vi "unphuck.vi"() -> ()   [LabVIEW 2009]
uses:
  <instrlib>/niScope/Controls/niScope vertical coupling.ctl
  Pulse Acquisition Method.ctl
  Pulse Queues.ctl
  <vilib>/Utility/file.llb/Write To Spreadsheet File (DBL).vi
  <instrlib>/niScope/Controls/niScope trigger slope.ctl
  <instrlib>/niScope/Controls/niScope trigger source.ctl
  <instrlib>/niScope/Configure/Trigger/niScope Configure Trigger Edge.vi
  <instrlib>/niScope/Acquire/Fetch/niScope Multi Fetch WDT.vi
panel:
  out "Number of Aquisitions":i32
  in  "Memory Repetition Period":dbl[unit]=0.025
  in  "Memory Acquisition Trigger Delay":dbl[unit] format="%.2f"
  out "Display Plot":bool
  in  "Get Reference Pulse":bool
  in  "Record Pulses":bool
  in  "Vertical range (0 to 10V)":dbl[unit]=0.01 caption="Vertical Range (V)" format="%.2f"
  in  "Desired Sample Rate":dbl[unit]=100000000.0 caption="Min. Sample Rate" step=1.0 format="%.2p"
  in  "Vertical coupling":T1 caption="Vertical Coupling" items=["AC", "DC", "Ground"]
  in  "Acquisition Time per Pulse":dbl[unit]=9.999999999999999e-06 format="%#.2g"
  out "Fetches Remaining":i32 caption="Number of Runs"
  out "Actual Sample Rate":dbl[unit]
  out "Number of Samples per Pulse":i32
  out "Acquisition Sequence":dbl[](graph)
  out "Total Acquired Time":dbl[unit]
  out "Total Number of Datapoints":i64=1000000
  out "Total Experiment Time":dbl[unit]
  in  "stop 2":bool
  in  "Number of Pulses":i32=40 caption="Number of Records"
  out "# Acquired":i32=100 caption="Number of Records Acquired"
  out "# Fetched":i32=100 caption="Number of Records Fetched"
  out "Data Directory":path
  out "Raw Phase, Trigger, Extracted Phase Data":path
  out "Quadrature Pulses File":path
  out "Reference Pulse File":path
  out "Shot Noise File":path
  out "Phase-Frequency Pairs":path
  out "Raman Measurement File Root":path
  # "Dependant Variables"
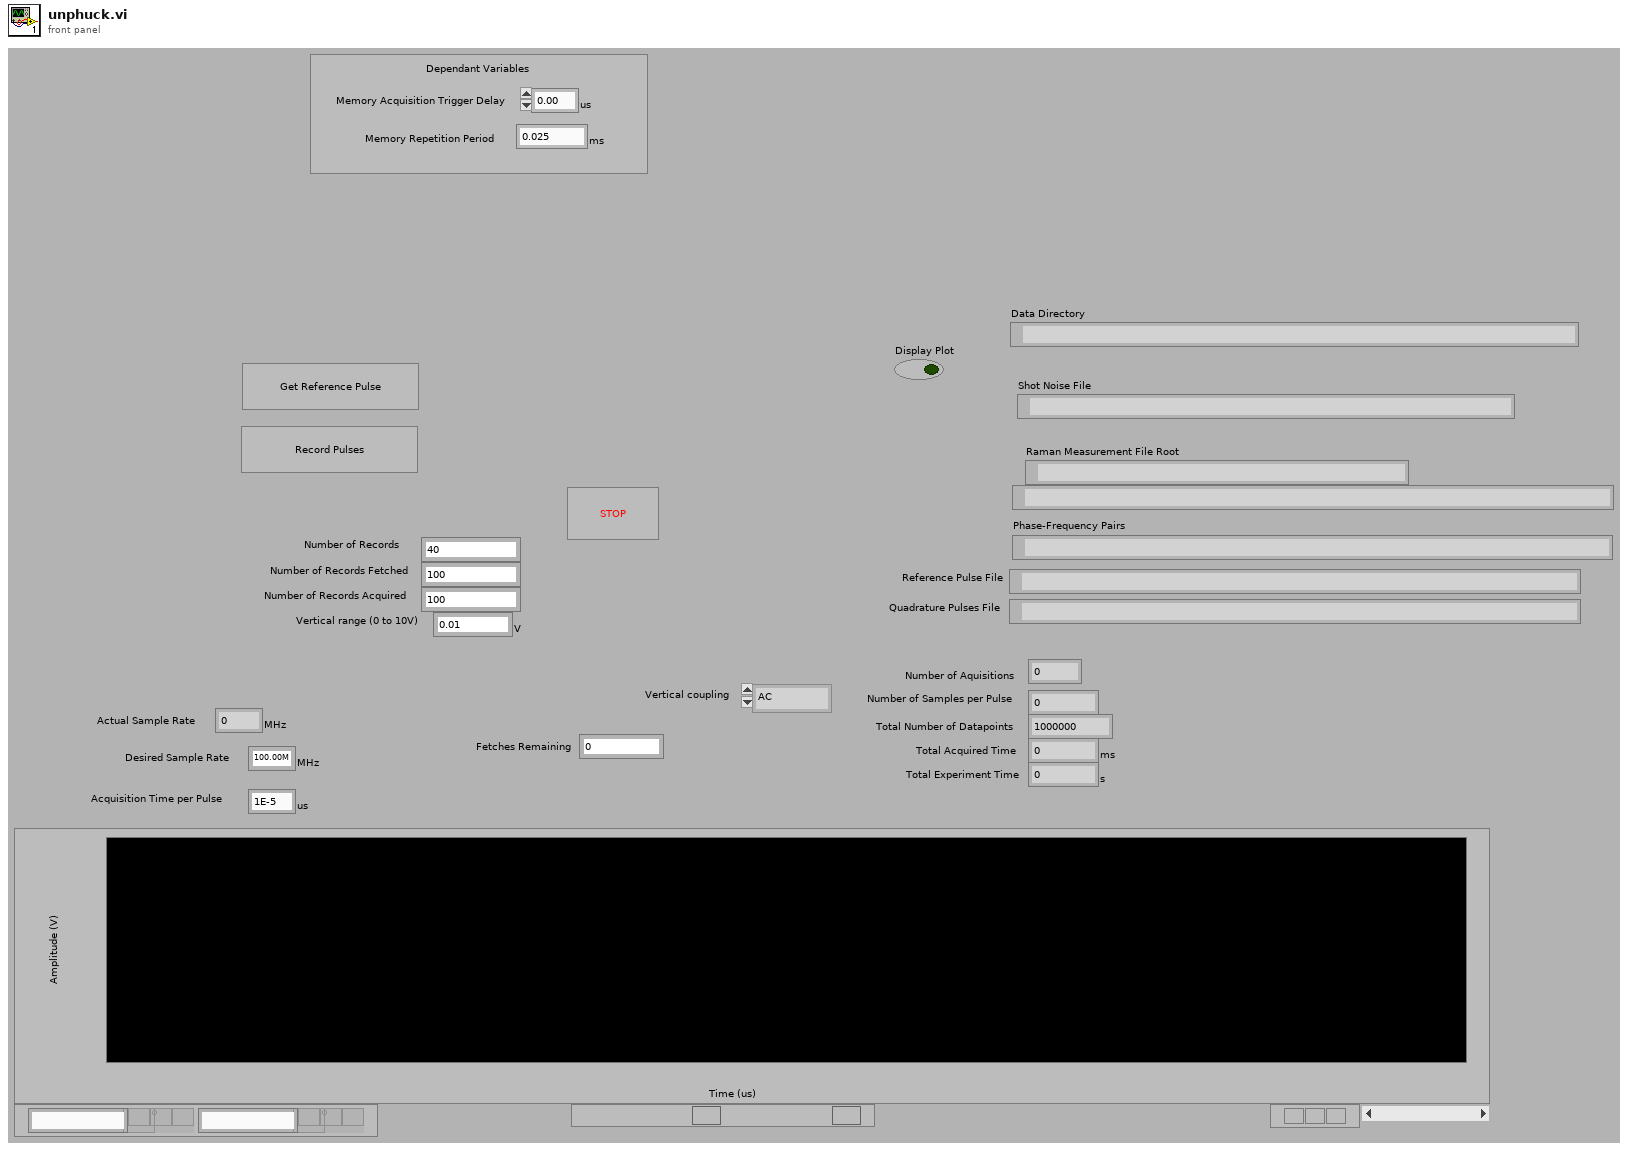
[diagram p1: front panel]
types:
  T1 = typedef "niScope vertical coupling.ctl" = i32
  T2 = typedef "Pulse Queues.ctl" = enum16{"Quadrature Queue", "Shot Queue"}
  T3 = enum16{"open", "replace", "create", "open or create", "replace or create", "replace or create with confirmation"}
  T4 = enum16{"open", "open or create", "create or replace", "create", "open (read-only)"}
  T5 = typedef "Pulse Acquisition Method.ctl" = enum16{"Initialize Batch Acqusition", "Initialize Monitor Acquisition", "Initialize Reference Acquisition", "Perform Batch Acquisition", "Perform Reference Acquisition", "Terminate Batch Acquisition", "Terminate Monitor Acqusition", "Terminate Reference Acquisition", "Standby"}
  T6 = typedef "niScope trigger source.ctl" = string
  T7 = typedef "niScope trigger slope.ctl" = i32
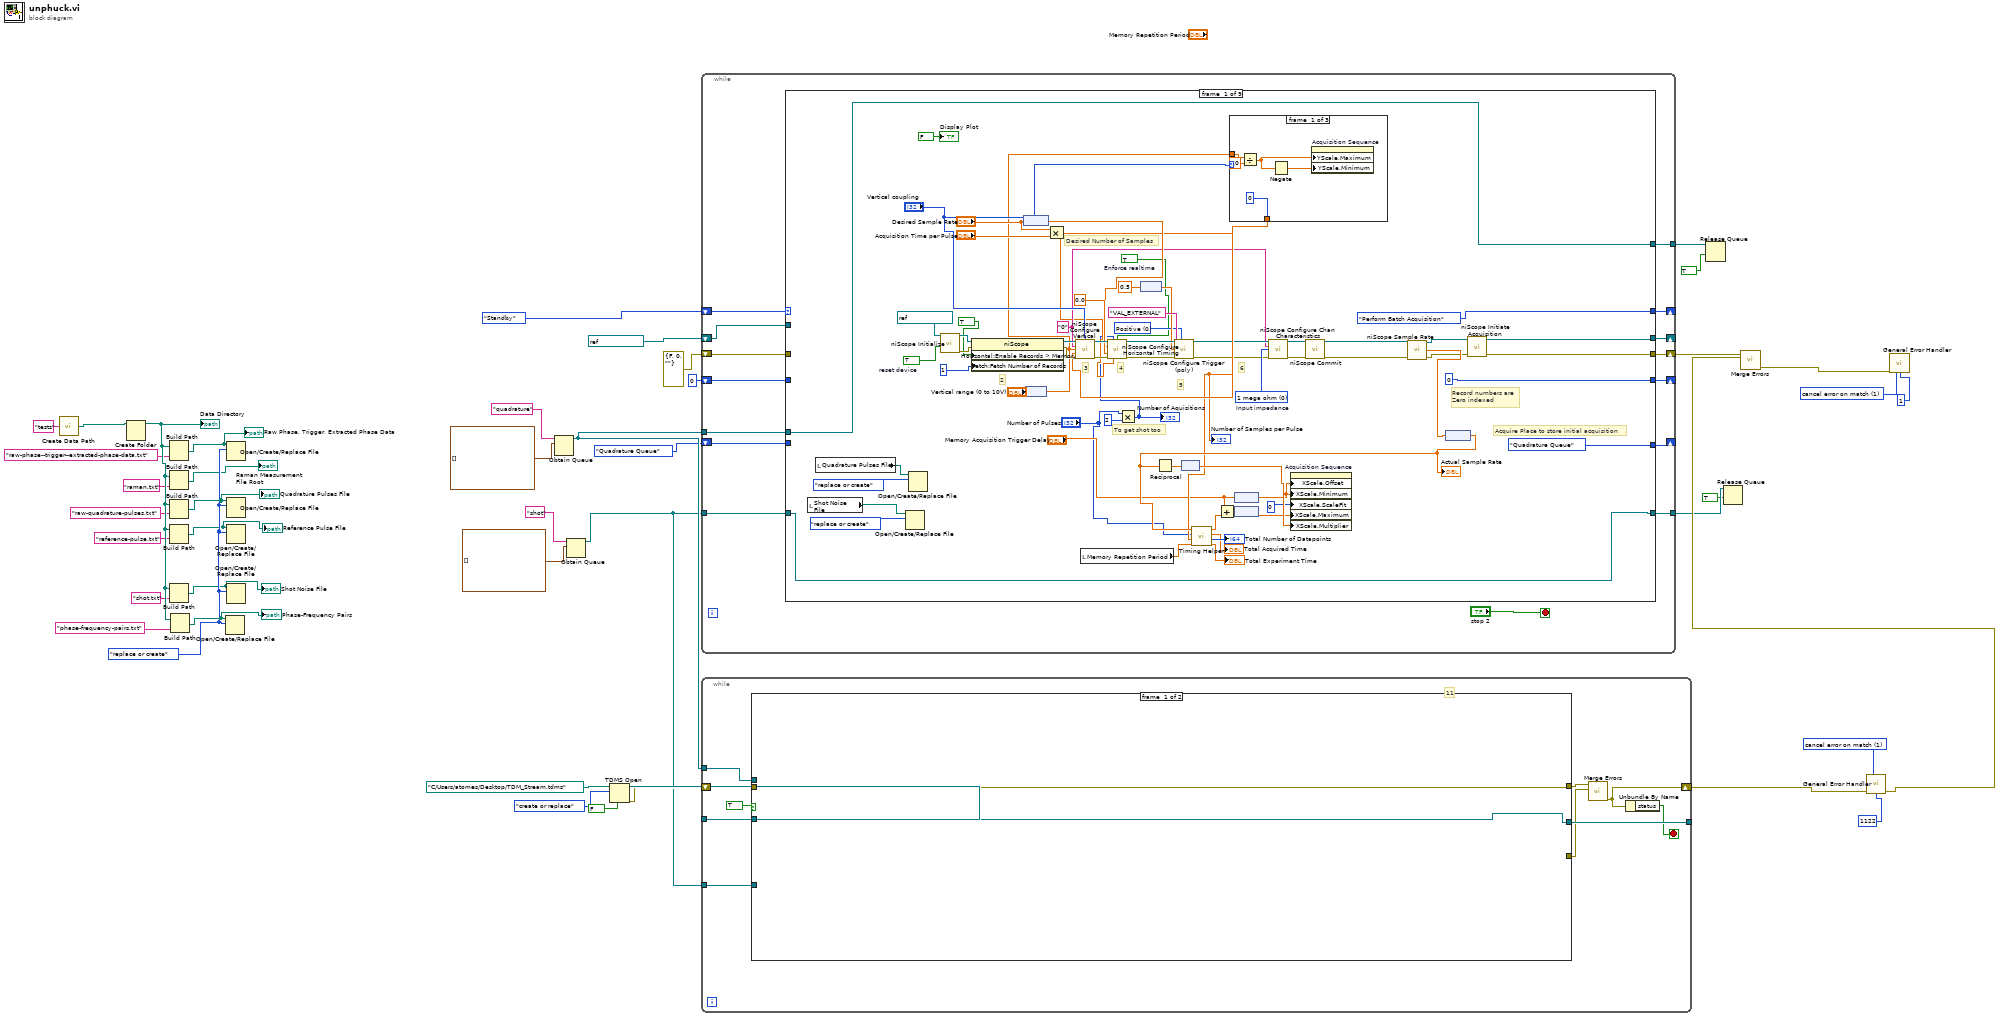
[diagram p0: block diagram]
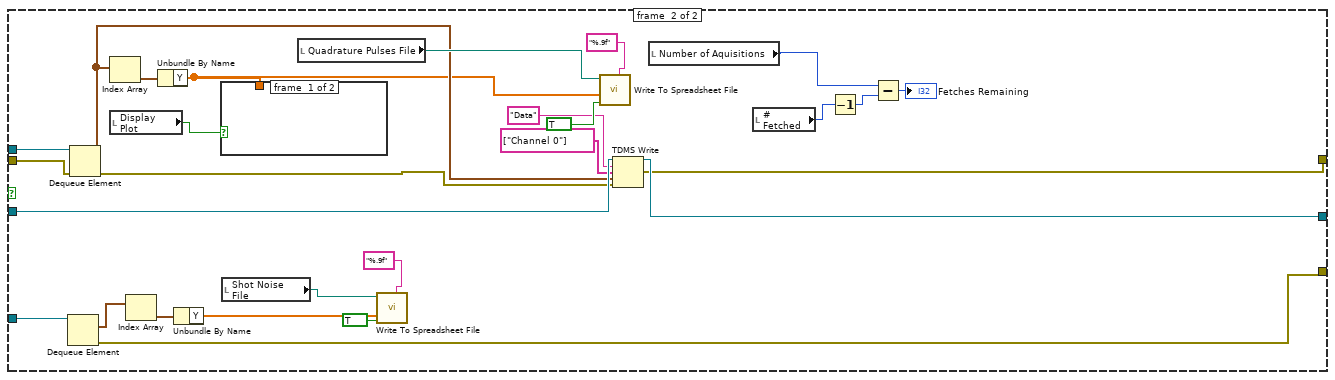
[diagram p2: hidden frame]
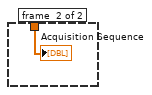
[diagram p3: hidden frame]
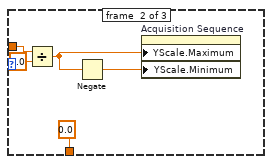
[diagram p4: hidden frame]
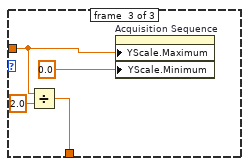
[diagram p5: hidden frame]
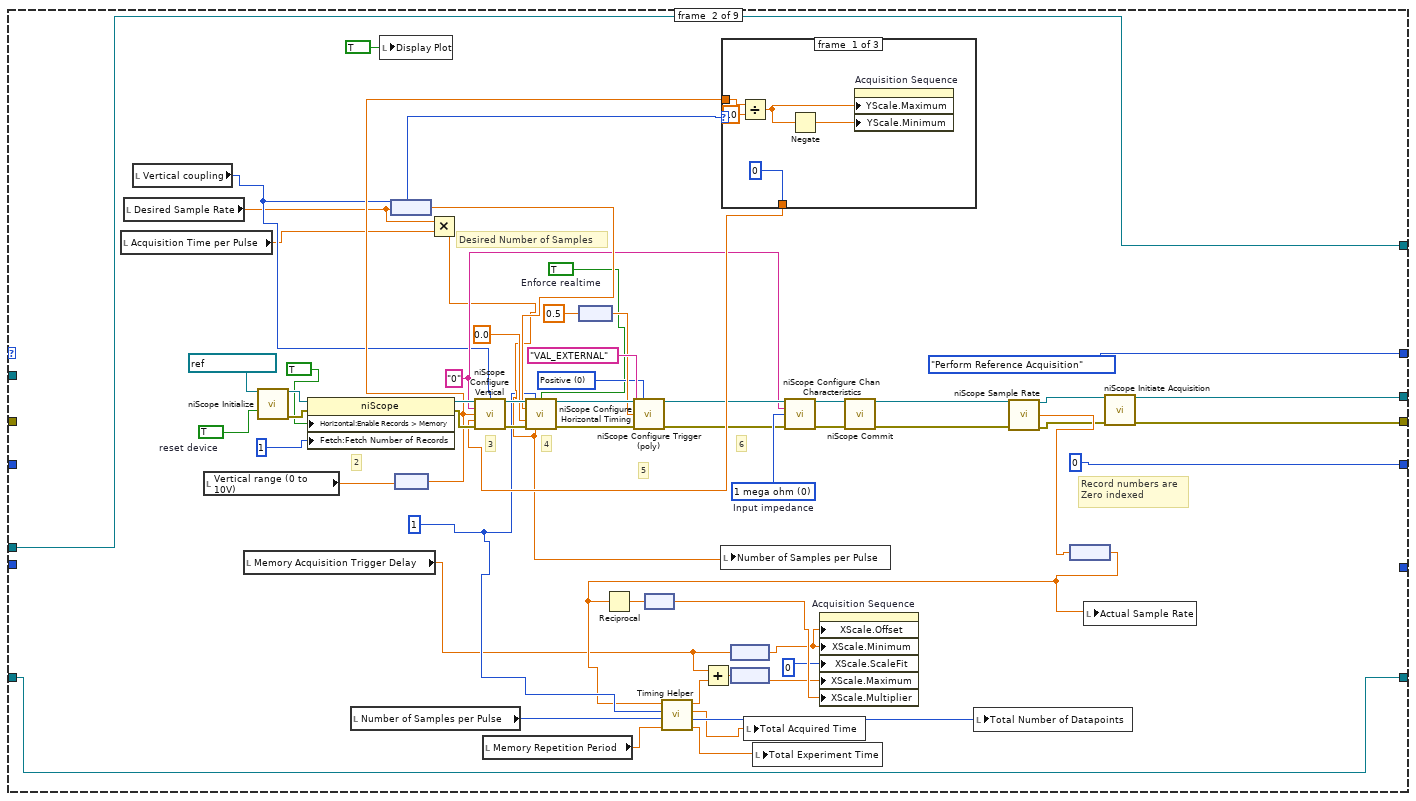
[diagram p6: hidden frame]
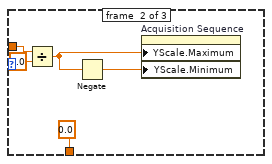
[diagram p7: hidden frame]
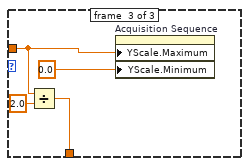
[diagram p8: hidden frame]
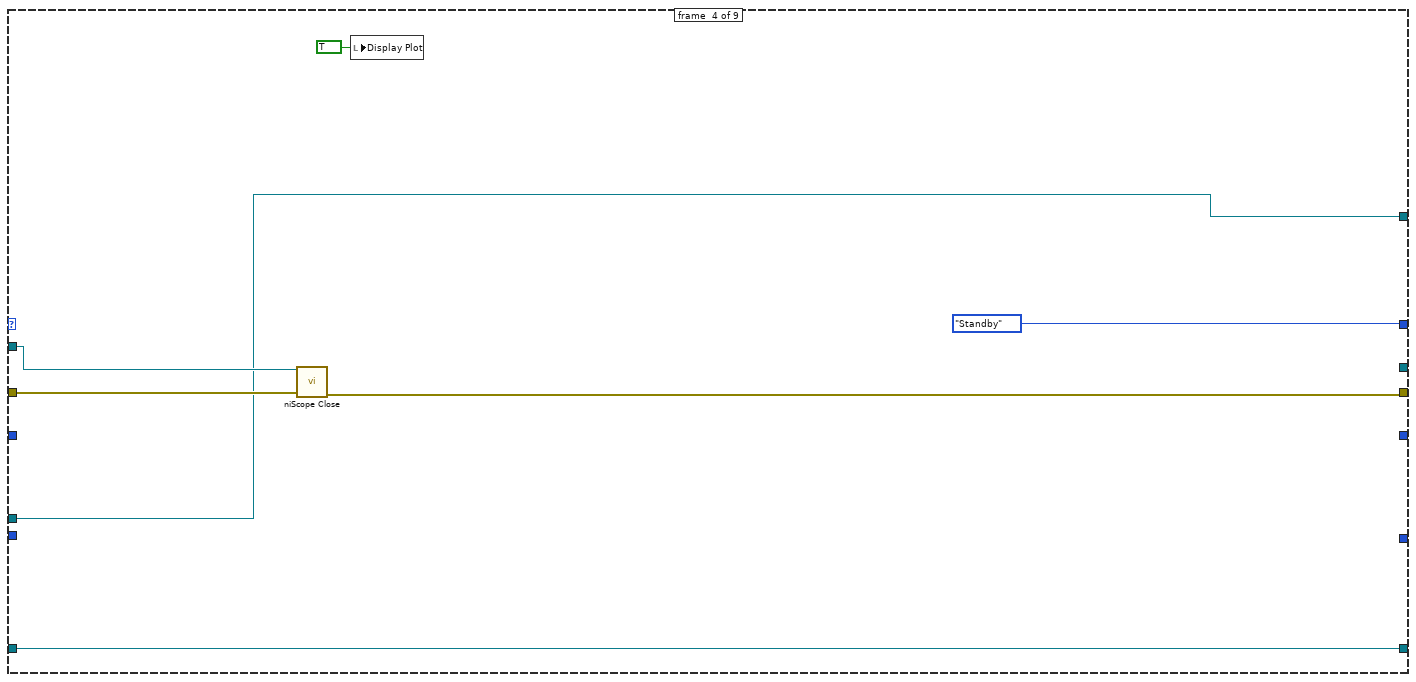
[diagram p10: hidden frame]
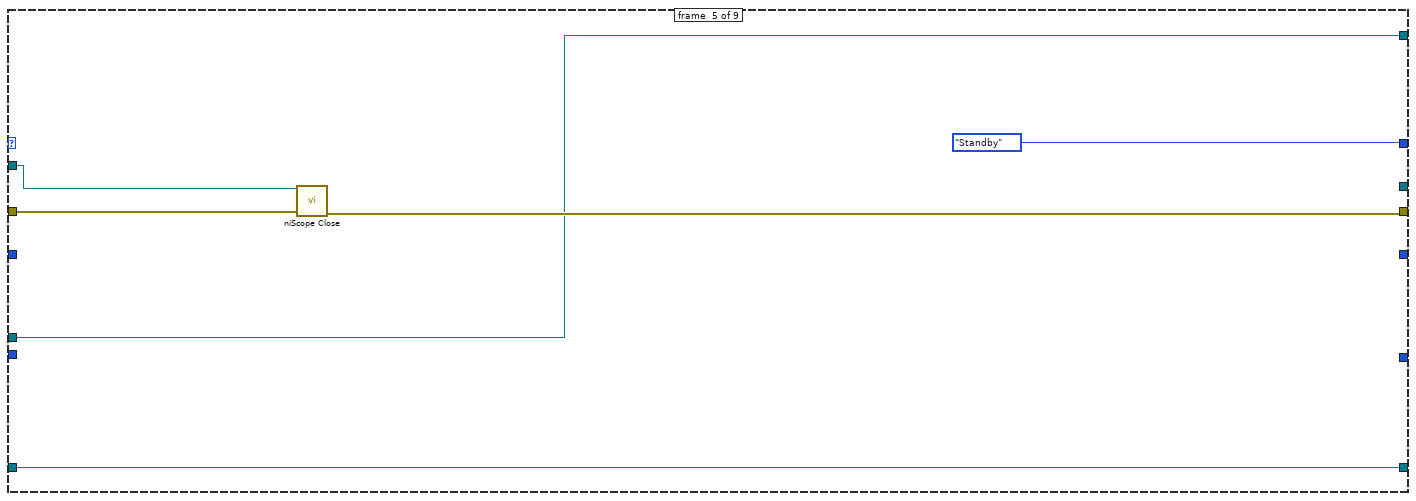
[diagram p11: hidden frame]
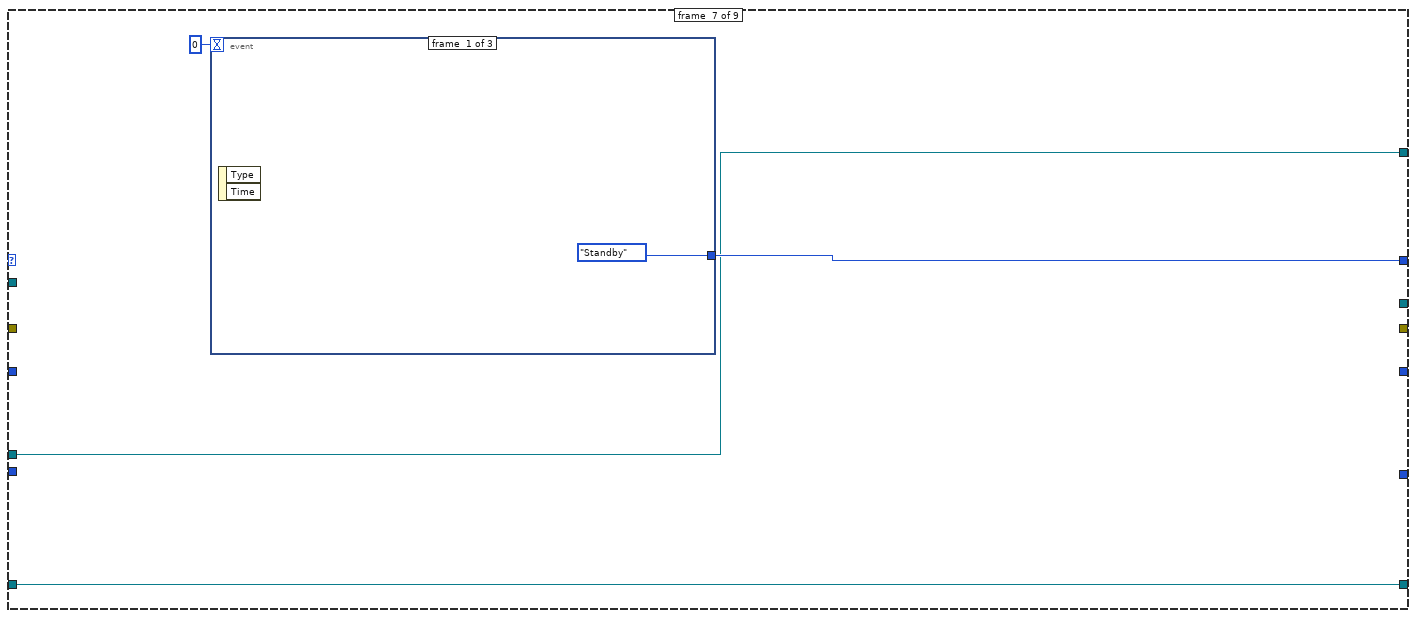
[diagram p13: hidden frame]
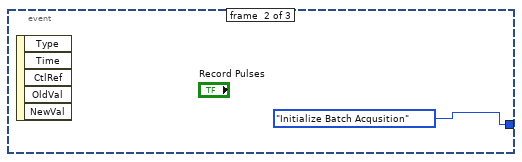
[diagram p14: hidden frame]
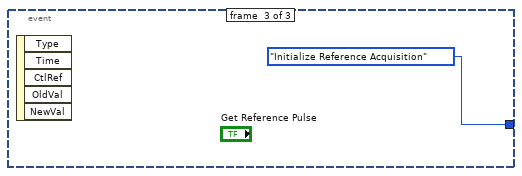
[diagram p15: hidden frame]
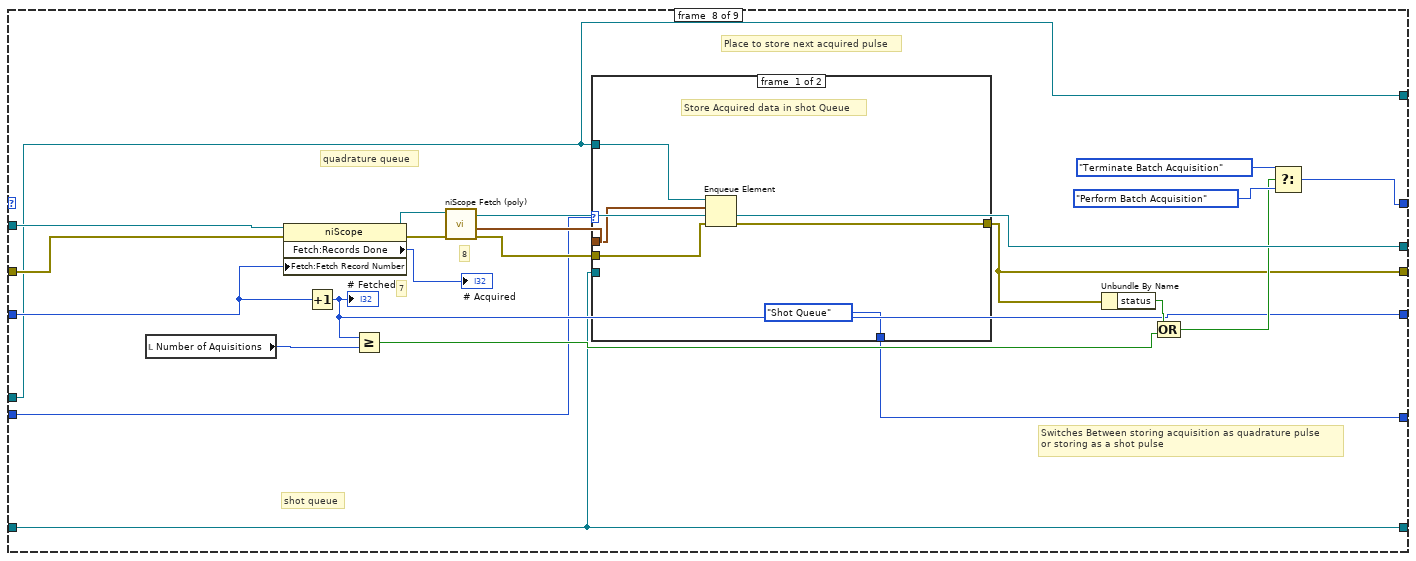
[diagram p16: hidden frame]
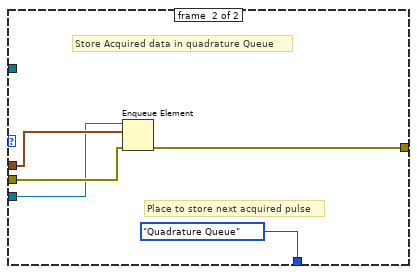
[diagram p17: hidden frame]
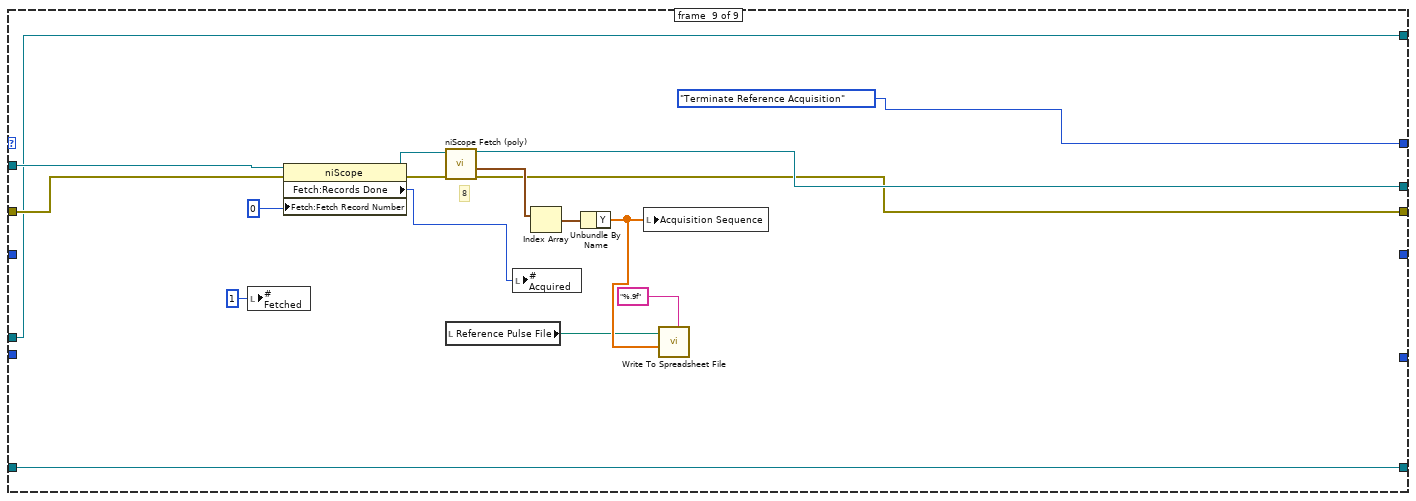
[diagram p18: hidden frame]
diagram:
  w7 = 1 items=["no exception", "cancel error on match", "set error on match"] ("[exception action] (none:0)")
  w12 = 1 items=["no exception", "cancel error on match", "set error on match"] ("[exception action] (none:0)")
  w35 = T3."replace or create" ("operation (0:open)")
  # "11"
  n1 = call "Create Data Path.vi"("Data Directory Name"="tests") -> ("appended path"=w24:path)
  n2 = Create Folder(path (use dialog)=w24) -> (created path=w33:path)  [unwired: 2 in, 2 out]
  "Data Directory" <- w33
  n3 = Build Path(base path=w33, name or relative path="raw-phase--trigger--extracted-phase-data.txt") -> (appended path=w26:path)
  "Raw Phase, Trigger, Extracted Phase Data" <- w26
  n4 = Build Path(base path=w33, name or relative path="raman.txt") -> (appended path=→"Raman Measurement File Root":path)
  n5 = Build Path(base path=w33, name or relative path="raw-quadrature-pulses.txt") -> (appended path=w28:path)
  "Quadrature Pulses File" <- w28
  n6 = Build Path(base path=w33, name or relative path="reference-pulse.txt") -> (appended path=w29:path)
  "Reference Pulse File" <- w29
  n7 = Build Path(base path=w33, name or relative path="shot.txt") -> (appended path=w30:path)
  "Shot Noise File" <- w30
  n8 = Build Path(base path=w33, name or relative path="phase-frequency-pairs.txt") -> (appended path=w34:path)
  "Phase-Frequency Pairs" <- w34
  n9 = Open/Create/Replace File(file path (use dialog)=w34, operation (0:open)=w35) -> ()  [unwired: 4 in, 3 out]
  n10 = Open/Create/Replace File(file path (use dialog)=w26, operation (0:open)=w35) -> ()  [unwired: 4 in, 3 out]
  n11 = Open/Create/Replace File(file path (use dialog)=w28, operation (0:open)=w35) -> ()  [unwired: 4 in, 3 out]
  n12 = Open/Create/Replace File(file path (use dialog)=w29, operation (0:open)=w35) -> ()  [unwired: 4 in, 3 out]
  n13 = Open/Create/Replace File(file path (use dialog)=w30, operation (0:open)=w35) -> ()  [unwired: 4 in, 3 out]
  n14 = Obtain Queue(name (unnamed)="quadrature", element data type=waveform(dbl)[] [] ("wfm")) -> (queue out=w36:refnum<queue>)  [unwired: 3 in, 2 out]
  n15 = Obtain Queue(name (unnamed)="shot", element data type=waveform(dbl)[] [] ("wfm")) -> (queue out=w4:refnum<queue>)  [unwired: 3 in, 2 out]
  n16 = TDMS Open(6:FALSE ("disable buffering (T)"), 10:T4."create or replace" ("operation"), 11:path "C:/Users/atomes/Desktop/TDM_Stream.tdms" ("selected path")) -> (0:w16:errorcluster, 3:w37:refnum<k34>)  [unwired: 3 in]
  n17 = while {
    tunnel: w36 -> [w51]
    tunnel: w37 -> [w54]
    tunnel: [w53] -> _
    shift-right: [w45] -> w10
    shift-left: w16 -> [w50]
    tunnel: w4 -> [w48]
    stop <- w52 stop-if-true
    n18 = case shown="True" TRUE {
      tunnel: w51 -> [_ w83]
      tunnel: w54 -> [w56 w82]
      tunnel: [w56 w81] -> w53
      tunnel: [w55 w79] -> w47
      tunnel: w50 -> [w55 w70]
      tunnel: w48 -> [_ w65]
      tunnel: [_ w58] -> w46
      frame #0 {
      }
      frame #1 {
        n19 = Dequeue Element(queue=w65) -> (element=w64:waveform(dbl)[], error out=w58:errorcluster)  [unwired: 2 in, 2 out]
        n20 = Dequeue Element(queue=w83, error in (no error)=w70) -> (element=w69:waveform(dbl)[], error out=w80:errorcluster)  [unwired: 1 in, 2 out]
        n21 = Index Array(array=w69) -> (element=w68:waveform(dbl))  [unwired: 1 in]
        n22 = local read "Display Plot"() -> (w66:bool)
        n23 = Index Array(array=w64) -> (element=w63:waveform(dbl))  [unwired: 1 in]
        n24 = Unbundle By Name(w68) -> ("Y"=w67:dbl[])
        n25 = Unbundle By Name(w63) -> ("Y"=w61:dbl[])
        n26 = case shown="True" w66 {
          tunnel: w67 -> [_ w84]
          frame #0 {
          }
          frame #1 {
            "Acquisition Sequence" <- w84
          }
        }
        n27 = local read "Shot Noise File"() -> (w59:path)
        n28 = local read "Quadrature Pulses File"() -> (w78:path)
        n29 = call-poly <vilib>:"Write To Spreadsheet File.vi"("format (%.3f)"="%.9f", "append to file? (new file:F)"=TRUE, "1D data"=w61, "file path (dialog if empty)"=w59) -> ()  [unwired: 2 in, 3 out]
        n30 = call-poly <vilib>:"Write To Spreadsheet File.vi"("format (%.3f)"="%.9f", "append to file? (new file:F)"=TRUE, "1D data"=w67, "file path (dialog if empty)"=w78) -> ()  [unwired: 2 in, 3 out]
        n31 = TDMS Write(0:w82, 5:"Data" ("group name in"), 7:string[] ["Channel 0"] ("channel name(s) in (Untitled)"), 9:w69, 11:w80) -> (4:w81:refnum<k34>, 15:w79:errorcluster)  [unwired: 1 in, 2 out]
        n32 = local read "Number of Aquisitions"() -> (w57:i32)
        n33 = local read "# Fetched"() -> (w72:i32)
        n34 = Decrement(x=w72) -> (x-1=w71:i32)
        n35 = Subtract(x=w57, y=w71) -> (x-y=→"Fetches Remaining":i32)
      }
    }
    n36 = call <vilib>:"Merge Errors.vi"("error in 2 (no error)"=w46, "error in 1 (no error)"=w47) -> ("error out"=w45:errorcluster)  [unwired: 2 in, 3 out]
    n37 = Unbundle By Name(w45) -> ("status"=w52:bool)
  }
  n38 = while {
    tunnel: w36 -> [w98]
    shift-right: [w97] -> _
    shift-left: refnum<k15> "Acquisition" ("instrument handle out") -> [w94]
    shift-right: [w96] -> w41
    shift-left: errorcluster {"status"=FALSE, "code"=0, "source"=""} ("error out") -> [w93]
    shift-right: [w95] -> _
    shift-left: Pulse_Acquisition_Method."Standby" ("Enum") -> [w99]
    shift-right: [w91] -> _
    shift-left: 0 -> [w92]
    tunnel: [w89] -> w15
    tunnel: w4 -> [w88]
    shift-right: [w86] -> _
    shift-left: Pulse_Queues."Quadrature Queue" ("Enum") -> [w87]
    tunnel: [w85] -> w2
    stop <- "stop 2" stop-if-true
    n39 = case shown="\"Initialize Batch Acqusition\", Default" w99 {
      tunnel: w98 -> [w113 w193 w253 w256 w262 w268 w271 w279 w315]
      tunnel: [w115 w195 _ _ _ _ _ w295 w322] -> w97
      tunnel: [w114 w194 _ w258 w264 _ _ w281 w313] -> w96
      tunnel: [Pulse_Acquisition_Method."Perform Batch Acquisition" ("Enum") Pulse_Acquisition_Method."Perform Reference Acquisition" ("Enum") _ Pulse_Acquisition_Method."Standby" ("Enum") Pulse_Acquisition_Method."Standby" ("Enum") _ w272 w287 Pulse_Acquisition_Method."Terminate Reference Acquisition" ("Enum")] -> w95
      tunnel: w94 -> [_ _ _ w260 w266 _ _ w297 w324]
      tunnel: w93 -> [_ _ _ w259 w265 _ _ w296 w323]
      tunnel: w92 -> [_ _ _ _ _ _ _ w285 _]
      tunnel: [0 0 _ _ _ _ _ w286 _] -> w91
      tunnel: [w113 w193 w253 w256 w262 w268 w271 w279 w315] -> w89
      tunnel: w88 -> [w103 w179 w252 w254 w261 w267 w269 w278 w308]
      tunnel: w87 -> [_ _ _ _ _ _ _ w280 _]
      tunnel: [Pulse_Queues."Quadrature Queue" ("Enum") _ _ _ _ _ _ w277 _] -> w86
      tunnel: [w103 w179 w252 w254 w261 w267 w269 w278 w308] -> w85
      frame #0 {
        w139 = T7 0 items=["Positive", "Negative"] ("trigger slope")
        w135 = TRUE  # Enforce realtime
        w147 = u32 0 items=["1 mega ohm", "75 ohms", "50 ohms"]  # Input impedance
        w134 = "0" ("channel name")
        w164 = TRUE  # reset device
        # "To get shot too"
        # "Acquire Place to store initial acquisition"
        # "Record numbers are\nZero indexed"
        # "Desired Number of Samples"
        # "6"
        # "5"
        # "4"
        # "3"
        # "2"
        n40 = local read "Shot Noise File"() -> (w105:path)
        n41 = local read "Quadrature Pulses File"() -> (w111:path)
        n42 = Open/Create/Replace File(file path (use dialog)=w105, operation (0:open)=T3."replace or create") -> ()  [unwired: 4 in, 3 out]
        n43 = Open/Create/Replace File(file path (use dialog)=w111, operation (0:open)=T3."replace or create") -> ()  [unwired: 4 in, 3 out]
        n44 = call <instrlib>:"niScope Initialize.vi"("resource name"=refnum<k15> "Acquisition", "reset device"=w164) -> ("instrument handle"=w162:refnum<k15>, "error out"=w161:errorcluster)  [unwired: 2 in, 10 out]
        n45 = property class="niScope"(reference=w162, error in=w161, "Horizontal:Enable Records > Memory"=TRUE ("Allow more records\nthan available memory?"), "Fetch:Fetch Number of Records"=1) -> (reference out=w160:refnum<k15>, error out=w159:errorcluster)
        n46 = node("Desired Sample Rate") -> (w136:dbl)
        n47 = node("Vertical range (0 to 10V)") -> (w141:dbl)
        n48 = Multiply(x="Desired Sample Rate", y="Acquisition Time per Pulse") -> (x*y=w108:dbl)
        "Number of Samples per Pulse" <- w108
        n49 = local read "Memory Repetition Period"() -> (w130:dbl[unit])
        n50 = Multiply(x="Number of Pulses", y=2) -> (x*y=w100:i32)
        "Number of Aquisitions" <- w100
        n51 = node(dbl[unit] 0.5 ("Trigger level")) -> (w140:dbl)
        n52 = case shown="0, Default" "Vertical coupling" {
          tunnel: w141 -> [w169 w174 w177]
          tunnel: [0 0.0 w175] -> w143
          frame #0 {
            n53 = Divide(x=w169, y=2.0) -> (x/y=w167:dbl)
            n54 = Negate(x=w167) -> (-x=w166:dbl)
            n55 = property on="Acquisition Sequence" class="WFGraph (strict)"("YScale.Maximum"=w167, "YScale.Minimum"=w166) -> ()  [unwired: 2 in, 2 out]
          }
          frame #1 {
            n56 = Divide(x=w174, y=2.0) -> (x/y=w172:dbl)
            n57 = Negate(x=w172) -> (-x=w171:dbl)
            n58 = property on="Acquisition Sequence" class="WFGraph (strict)"("YScale.Maximum"=w172, "YScale.Minimum"=w171) -> ()  [unwired: 2 in, 2 out]
          }
          frame #2 {
            n59 = Divide(x=w177, y=2.0) -> (x/y=w175:dbl)
            n60 = property on="Acquisition Sequence" class="WFGraph (strict)"("YScale.Maximum"=w177, "YScale.Minimum"=0.0 ("Y Scale.Range:Minimum")) -> ()  [unwired: 2 in, 2 out]
          }
        }
        n61 = call <instrlib>:"niScope Configure Vertical.vi"("instrument handle"=w160, "vertical coupling"="Vertical coupling", "channels"=w134, "vertical range"=w141, "vertical offset"=w143, "error in"=w159) -> ("instrument handle out"=w157:refnum<k15>, "error out"=w156:errorcluster)  [unwired: 2 in, 6 out]
        n62 = call <instrlib>:"niScope Configure Horizontal Timing.vi"("instrument handle"=w157, "number of records"=w100, "enforce realtime"=w135, "min sample rate"=w136, "reference position"=0.0, "error in"=w156, "min record length"=w108) -> ("instrument handle out"=w155:refnum<k15>, "error out"=w154:errorcluster)  [unwired: 7 out]
        n63 = call-poly <instrlib>:"niScope Configure Trigger (poly).vi"("instrument handle"=w155, "trigger slope"=w139, "trigger source"=T6 "VAL_EXTERNAL", "trigger level"=w140, "error in"=w154) -> ("instrument handle out"=w138:refnum<k15>, "error out"=w137:errorcluster)  [unwired: 3 in, 6 out]
        n64 = node("Memory Acquisition Trigger Delay") -> (w129:dbl)
        n65 = call <instrlib>:"niScope Configure Chan Characteristics.vi"("instrument handle"=w138, "channels"=w134, "input impedance"=w147, "error in"=w137) -> ("instrument handle out"=w121:refnum<k15>, "error out"=w120:errorcluster)  [unwired: 1 in, 9 out]
        n66 = call <instrlib>:"niScope Commit.vi"("instrument handle"=w121, "error in"=w120) -> ("instrument handle out"=w119:refnum<k15>, "error out"=w118:errorcluster)  [unwired: 12 in]
        n67 = call <instrlib>:"niScope Sample Rate.vi"("instrument handle"=w119, "error in"=w118) -> ("instrument handle out"=w116:refnum<k15>, "actual sample rate"=w133:dbl, "error out"=w117:errorcluster)  [unwired: 11 out]
        n68 = node(w133) -> (w109:dbl[unit])
        "Actual Sample Rate" <- w109
        n69 = Reciprocal(x=w109) -> (1/x=w131:dbl[unit])
        n70 = node(w131) -> (w132:dbl)
        n71 = call "Timing Helper.vi"("Repetition Period"=w130, "Number of points per run"=w108, "Number of runs"="Number of Pulses", "Sample rate"=w109) -> ("Total Experiment Time"=→"Total Experiment Time":dbl[unit], "Total Number of Datapoints"=→"Total Number of Datapoints":i64, "Total Acquired Time"=→"Total Acquired Time":dbl[unit], "Acquisition Time per Run"=w122:dbl[unit])
        n72 = Add(x="Memory Acquisition Trigger Delay", y=w122) -> (x+y=w126:dbl[unit])
        n73 = node(w126) -> (w128:dbl)
        n74 = property on="Acquisition Sequence" class="WFGraph (strict)"("XScale.Offset"=w129, "XScale.Minimum"=w129, "XScale.ScaleFit"=u8 0 ("X Scale.Scale Fit"), "XScale.Maximum"=w128, "XScale.Multiplier"=w132) -> ()  [unwired: 2 in, 2 out]
        n75 = call <instrlib>:"niScope Initiate Acquisition.vi"("instrument handle"=w116, "error in"=w117) -> ("instrument handle out"=w115:refnum<k15>, "error out"=w114:errorcluster)  [unwired: 12 out]
        "Display Plot" <- FALSE
      }
      frame #1 {
        w184 = 1 ("number of records")
        w216 = T7 0 items=["Positive", "Negative"] ("trigger slope")
        w212 = TRUE  # Enforce realtime
        w221 = u32 0 items=["1 mega ohm", "75 ohms", "50 ohms"]  # Input impedance
        w211 = "0" ("channel name")
        w237 = TRUE  # reset device
        # "Record numbers are\nZero indexed"
        # "Desired Number of Samples"
        # "6"
        # "5"
        # "4"
        # "3"
        # "2"
        n76 = local read "Acquisition Time per Pulse"() -> (w190:dbl[unit])
        n77 = local read "Desired Sample Rate"() -> (w191:dbl[unit])
        n78 = local read "Vertical coupling"() -> (w192:T1)
        n79 = local read "Vertical range (0 to 10V)"() -> (w189:dbl[unit])
        n80 = local read "Memory Acquisition Trigger Delay"() -> (w181:dbl[unit])
        n81 = call <instrlib>:"niScope Initialize.vi"("resource name"=refnum<k15> "Acquisition", "reset device"=w237) -> ("instrument handle"=w235:refnum<k15>, "error out"=w234:errorcluster)  [unwired: 2 in, 10 out]
        n82 = property class="niScope"(reference=w235, error in=w234, "Horizontal:Enable Records > Memory"=TRUE ("Allow more records\nthan available memory?"), "Fetch:Fetch Number of Records"=1) -> (reference out=w233:refnum<k15>, error out=w232:errorcluster)
        n83 = local read "Number of Samples per Pulse"() -> (w202:i32)
        n84 = local write "Display Plot"(TRUE ("Display Plot")) -> ()
        n85 = node(w191) -> (w213:dbl)
        n86 = node(w189) -> (w218:dbl)
        n87 = Multiply(x=w191, y=w190) -> (x*y=w185:dbl)
        n88 = local read "Memory Repetition Period"() -> (w207:dbl[unit])
        n89 = node(dbl[unit] 0.5 ("Trigger level")) -> (w217:dbl)
        n90 = local write "Number of Samples per Pulse"(w185) -> ()
        n91 = case shown="0, Default" w192 {
          tunnel: w218 -> [w242 w247 w250]
          tunnel: [0 0.0 w248] -> w219
          frame #0 {
            n92 = Divide(x=w242, y=2.0) -> (x/y=w240:dbl)
            n93 = Negate(x=w240) -> (-x=w239:dbl)
            n94 = property on="Acquisition Sequence" class="WFGraph (strict)"("YScale.Maximum"=w240, "YScale.Minimum"=w239) -> ()  [unwired: 2 in, 2 out]
          }
          frame #1 {
            n95 = Divide(x=w247, y=2.0) -> (x/y=w245:dbl)
            n96 = Negate(x=w245) -> (-x=w244:dbl)
            n97 = property on="Acquisition Sequence" class="WFGraph (strict)"("YScale.Maximum"=w245, "YScale.Minimum"=w244) -> ()  [unwired: 2 in, 2 out]
          }
          frame #2 {
            n98 = Divide(x=w250, y=2.0) -> (x/y=w248:dbl)
            n99 = property on="Acquisition Sequence" class="WFGraph (strict)"("YScale.Maximum"=w250, "YScale.Minimum"=0.0 ("Y Scale.Range:Minimum")) -> ()  [unwired: 2 in, 2 out]
          }
        }
        n100 = call <instrlib>:"niScope Configure Vertical.vi"("instrument handle"=w233, "vertical coupling"=w192, "channels"=w211, "vertical range"=w218, "vertical offset"=w219, "error in"=w232) -> ("instrument handle out"=w230:refnum<k15>, "error out"=w229:errorcluster)  [unwired: 2 in, 6 out]
        n101 = call <instrlib>:"niScope Configure Horizontal Timing.vi"("instrument handle"=w230, "number of records"=w184, "enforce realtime"=w212, "min sample rate"=w213, "reference position"=0.0, "error in"=w229, "min record length"=w185) -> ("instrument handle out"=w228:refnum<k15>, "error out"=w227:errorcluster)  [unwired: 7 out]
        n102 = call-poly <instrlib>:"niScope Configure Trigger (poly).vi"("instrument handle"=w228, "trigger slope"=w216, "trigger source"=T6 "VAL_EXTERNAL", "trigger level"=w217, "error in"=w227) -> ("instrument handle out"=w215:refnum<k15>, "error out"=w214:errorcluster)  [unwired: 3 in, 6 out]
        n103 = node(w181) -> (w180:dbl)
        n104 = call <instrlib>:"niScope Configure Chan Characteristics.vi"("instrument handle"=w215, "channels"=w211, "input impedance"=w221, "error in"=w214) -> ("instrument handle out"=w201:refnum<k15>, "error out"=w200:errorcluster)  [unwired: 1 in, 9 out]
        n105 = call <instrlib>:"niScope Commit.vi"("instrument handle"=w201, "error in"=w200) -> ("instrument handle out"=w199:refnum<k15>, "error out"=w198:errorcluster)  [unwired: 12 in]
        n106 = call <instrlib>:"niScope Sample Rate.vi"("instrument handle"=w199, "error in"=w198) -> ("instrument handle out"=w196:refnum<k15>, "actual sample rate"=w210:dbl, "error out"=w197:errorcluster)  [unwired: 11 out]
        n107 = node(w210) -> (w182:dbl[unit])
        n108 = Reciprocal(x=w182) -> (1/x=w208:dbl[unit])
        n109 = node(w208) -> (w209:dbl)
        n110 = call "Timing Helper.vi"("Repetition Period"=w207, "Number of points per run"=w202, "Number of runs"=w184, "Sample rate"=w182) -> ("Total Experiment Time"=w186:dbl[unit], "Total Number of Datapoints"=w188:i64, "Total Acquired Time"=w187:dbl[unit], "Acquisition Time per Run"=w203:dbl[unit])
        n111 = Add(x=w181, y=w203) -> (x+y=w204:dbl[unit])
        n112 = node(w204) -> (w206:dbl)
        n113 = local write "Total Acquired Time"(w187) -> ()
        n114 = local write "Total Experiment Time"(w186) -> ()
        n115 = property on="Acquisition Sequence" class="WFGraph (strict)"("XScale.Offset"=w180, "XScale.Minimum"=w180, "XScale.ScaleFit"=u8 0 ("X Scale.Scale Fit"), "XScale.Maximum"=w206, "XScale.Multiplier"=w209) -> ()  [unwired: 2 in, 2 out]
        n116 = local write "Total Number of Datapoints"(w188) -> ()
        n117 = local write "Actual Sample Rate"(w182) -> ()
        n118 = call <instrlib>:"niScope Initiate Acquisition.vi"("instrument handle"=w196, "error in"=w197) -> ("instrument handle out"=w195:refnum<k15>, "error out"=w194:errorcluster)  [unwired: 12 out]
      }
      frame #2 {
      }
      frame #3 {
        n119 = call <instrlib>:"niScope Close.vi"("instrument handle"=w260, "error in"=w259) -> ("error out"=w258:errorcluster)  [unwired: 13 out]
        n120 = local write "Display Plot"(TRUE ("Display Plot")) -> ()
      }
      frame #4 {
        n121 = call <instrlib>:"niScope Close.vi"("instrument handle"=w266, "error in"=w265) -> ("error out"=w264:errorcluster)  [unwired: 13 out]
      }
      frame #5 {
      }
      frame #6 {
        n122 = event shown="[2] \"Get Reference Pulse\": Value Change" {
          selector: _ -> [_ _ _]
          dyn-events: _ -> [_ _ _]
          timeout: 0 -> [_ _ _]
          tunnel: [Pulse_Acquisition_Method."Standby" ("Enum") Pulse_Acquisition_Method."Initialize Batch Acqusition" ("Enum") Pulse_Acquisition_Method."Initialize Reference Acquisition" ("Enum")] -> w272
          event #0 {
            n123 = event-data() -> ()  [unwired: 1 in, 2 out]
          }
          event #1 {
            n124 = event-data() -> ()  [unwired: 1 in, 5 out]
          }
          event #2 {
            n125 = event-data() -> ()  [unwired: 1 in, 5 out]
          }
        }
      }
      frame #7 {
        # "Place to store next acquired pulse"
        # "shot queue"
        # "quadrature queue"
        # "Switches Between storing acquisition as quadrature pulse\nor storing as a shot pulse"
        # "8"
        # "7"
        n126 = local read "Number of Aquisitions"() -> (w276:i32)
        n127 = property class="niScope"(reference=w297, error in=w296, "Fetch:Fetch Record Number"=w285) -> (reference out=w289:refnum<k15>, error out=w292:errorcluster, "Fetch:Records Done"=→"# Acquired":i32)
        n128 = Increment(x=w285) -> (x+1=w286:i32)
        "# Fetched" <- w286
        n129 = Greater Or Equal?(x=w286, y=w276) -> (x >= y?=w291:bool)
        n130 = call-poly <instrlib>:"niScope Fetch (poly).vi"("error in"=w292, "instrument handle"=w289) -> ("error out"=w282:errorcluster, "wfm"=w283:waveform(dbl)[], "instrument handle out"=w295:refnum<k15>)  [unwired: 4 in, 3 out]
        n131 = case shown="\"Shot Queue\"" w280 {
          tunnel: w283 -> [w301 w306]
          tunnel: w278 -> [_ w304]
          tunnel: [w302 w307] -> w281
          tunnel: w282 -> [w300 w305]
          tunnel: w279 -> [w299 _]
          tunnel: [Pulse_Queues."Shot Queue" ("Enum") Pulse_Queues."Quadrature Queue" ("Enum")] -> w277
          frame #0 {
            # "Store Acquired data in shot Queue"
            n132 = Enqueue Element(queue=w299, element=w301, error in (no error)=w300) -> (error out=w302:errorcluster)  [unwired: 3 out]
          }
          frame #1 {
            # "Place to store next acquired pulse"
            # "Store Acquired data in quadrature Queue"
            n133 = Enqueue Element(queue=w304, element=w306, error in (no error)=w305) -> (error out=w307:errorcluster)  [unwired: 3 out]
          }
        }
        n134 = Unbundle By Name(w281) -> ("status"=w290:bool)
        n135 = Compound Arithmetic op=OR(w290, w291) -> (w288:bool)
        n136 = Select(t=Pulse_Acquisition_Method."Terminate Batch Acquisition" ("Enum"), s=w288, f=Pulse_Acquisition_Method."Perform Batch Acquisition" ("Enum")) -> (s? t:f=w287:T5)
      }
      frame #8 {
        # "8"
        n137 = local write "# Fetched"(1 ("# Fetched")) -> ()
        n138 = property class="niScope"(reference=w324, error in=w323, "Fetch:Fetch Record Number"=0) -> (reference out=w320:refnum<k15>, error out=w321:errorcluster, "Fetch:Records Done"=w309:i32)
        n139 = call-poly <instrlib>:"niScope Fetch (poly).vi"("error in"=w321, "instrument handle"=w320) -> ("error out"=w313:errorcluster, "wfm"=w314:waveform(dbl)[], "instrument handle out"=w322:refnum<k15>)  [unwired: 4 in, 3 out]
        n140 = local read "Reference Pulse File"() -> (w310:path)
        n141 = local write "# Acquired"(w309) -> ()
        n142 = Index Array(array=w314) -> (element=w316:waveform(dbl))  [unwired: 1 in]
        n143 = Unbundle By Name(w316) -> ("Y"=w311:dbl[])
        n144 = local write "Acquisition Sequence"(w311) -> ()
        n145 = call-poly <vilib>:"Write To Spreadsheet File.vi"("format (%.3f)"="%.9f", "1D data"=w311, "file path (dialog if empty)"=w310) -> ()  [unwired: 3 in, 3 out]
      }
    }
  }
  n146 = Release Queue(queue=w15, force destroy? (F)=TRUE) -> ()  [unwired: 1 in, 3 out]
  n147 = Release Queue(queue=w2, force destroy? (F)=TRUE) -> ()  [unwired: 1 in, 3 out]
  n148 = call <vilib>:"General Error Handler.vi"("error in (no error)"=w10, "[exception action] (none:0)"=w7, "[exception code]"=1122 ("[error code] (0)")) -> ("error out"=w9:errorcluster)  [unwired: 8 in, 4 out]
  n149 = call <vilib>:"Merge Errors.vi"("error in 2 (no error)"=w9, "error in 1 (no error)"=w41) -> ("error out"=w13:errorcluster)  [unwired: 2 in, 3 out]
  n150 = call <vilib>:"General Error Handler.vi"("error in (no error)"=w13, "[exception action] (none:0)"=w12, "[exception code]"=1 ("[error code] (0)")) -> ()  [unwired: 8 in, 5 out]
